vi "自定义模板.vi"() -> ()   [LabVIEW 2016]
uses:
  <vilib>/vision/Image Controls.llb/IMAQ Image.ctl
  <vilib>/vision/driver/IMAQdx.llb/IMAQdx Buffer Number Mode.ctl
  <vilib>/userdefined/High Color/IMAQdx.ctl
  <vilib>/vision/driver/IMAQdx.llb/IMAQdx Acquisition Mode.ctl
  <vilib>/vision/driver/NI_Vision_Acquisition_Software.lvlib
  <vilib>/vision/NI_Vision_Development_Module.lvlib
panel:
  in  "选项卡控件":enum32{"选项卡 1"}(tab)
  in  "导入图片":bool
  in  "保存按钮":bool
  in  "Stop":bool
  out "模板":T1(plugin-control)
  out "原图":T1(plugin-control)
  out "字符串":string="等待PLC端触发信号"
  in  "PLC触发拍照":bool
  # "自定义模板界面"
  # "1、点击导入图片选择原图.PNG"
  # "2、在原图中按住鼠标左键框选自定义模板（框选中间的圆形孔），选择完成后松开左键"
  # "3、模板中显示框选的模板，如不满意重新第二步骤"
  # "4、点击保存，在对话框中选择模板.PNG进行覆盖"
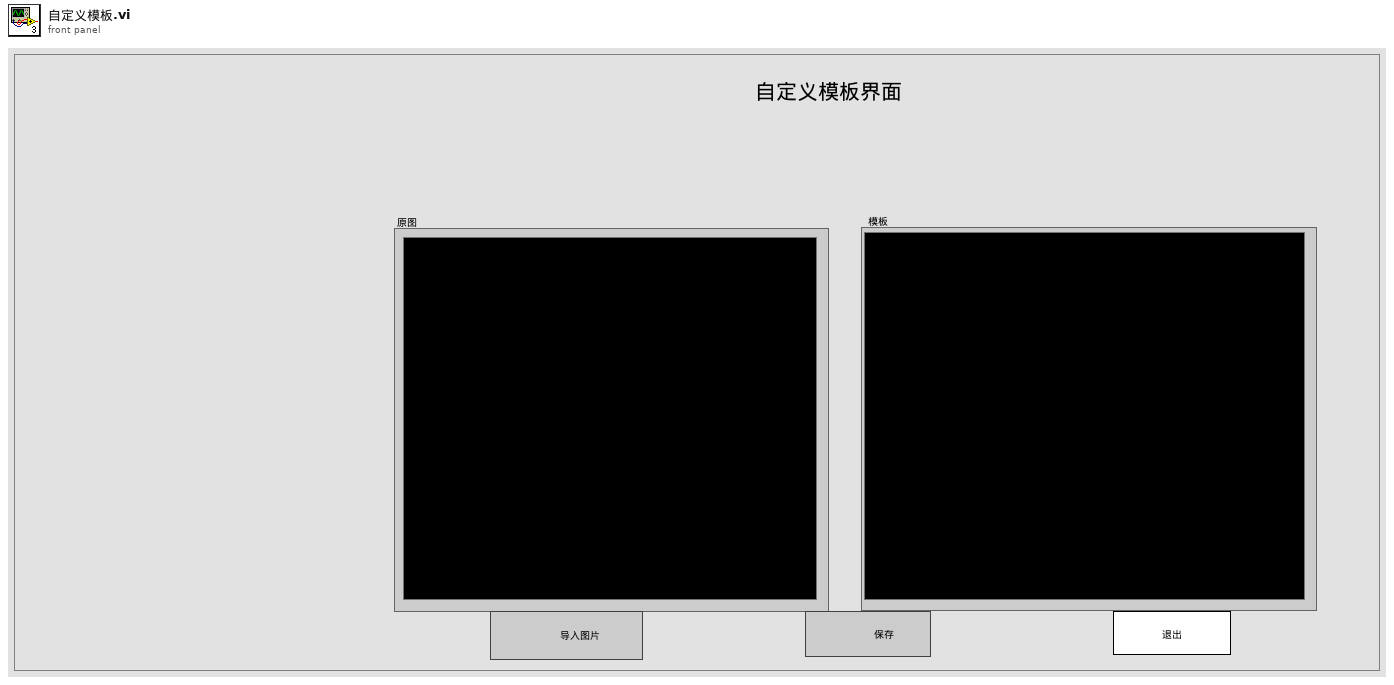
[diagram p1: front panel]
types:
  T1 = typedef "IMAQ Image.ctl" = refnum<image>
  T2 = typedef "建模板.ctl" = enum16{"等待", "拍照", "导入图片", "画模板", "保存模板", "左移", "右移", "上移", "下移", "旋转", "左右拉伸", "上下拉伸", "刷新图片", "保存参数", "退出"}
  T3 = enum8{"Enabled", "Disabled", "Disabled and Grayed Out"}
  T4 = typedef "Image Type" = u32
  T5 = cluster{"Zoom Tool":bool, "Selection Tool":bool, "Pan Tool":bool, "Point Tool":bool, "Line Tool":bool, "Rectangle Tool":bool, "Rotated Rectangle Tool":bool, "Polyline Tool":bool, "Polygon Tool":bool, "Freehand Tool":bool, "Closed Freehand Tool":bool, "Ellipse Tool":bool, "Annulus Tool":bool}
  T6 = typedef "NI_Vision_Acquisition_Software.lvlib/IMAQdx Acquisition Mode.ctl" = enum32{"One Shot", "Continuous"}
  T7 = typedef "IMAQdx.ctl" = refnum<k21>
  T8 = typedef "NI_Vision_Acquisition_Software.lvlib/IMAQdx Buffer Number Mode.ctl" = enum32{"Next", "Last", "Buffer Number", "Every", "Last New"}
  T9 = cluster{"Match Mode":u16, "Number of Matches Requested":i32, "Minimum Match Score":sgl, "SubPixel Accuracy":bool, "Rotation Angle Ranges":cluster{"Start":sgl, "End":sgl}[], "Show Search Area":bool, "Show Result":bool}
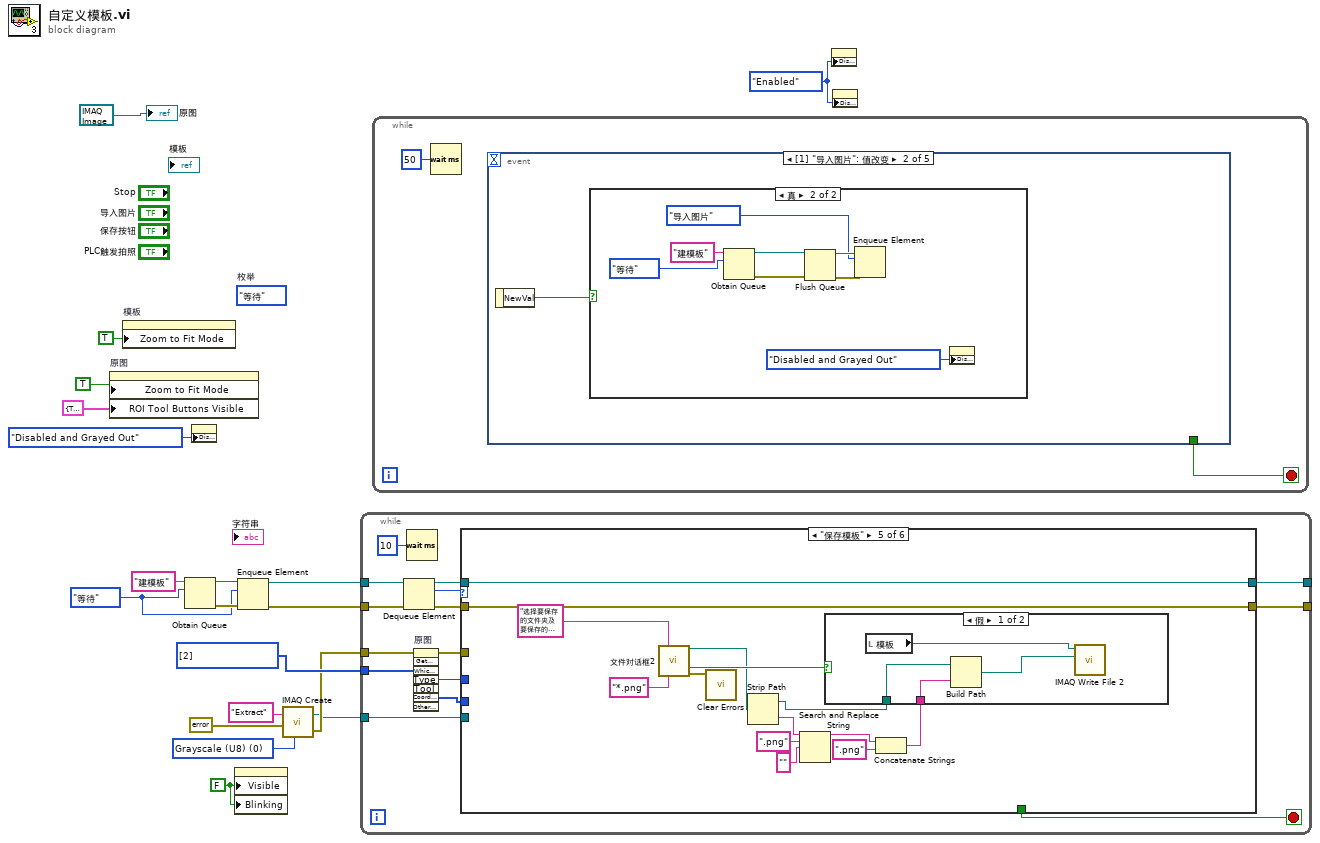
[diagram p0: block diagram]
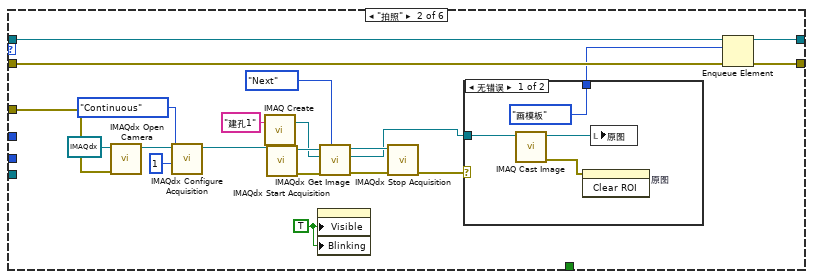
[diagram p3: hidden frame]
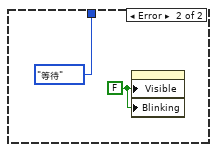
[diagram p4: hidden frame]
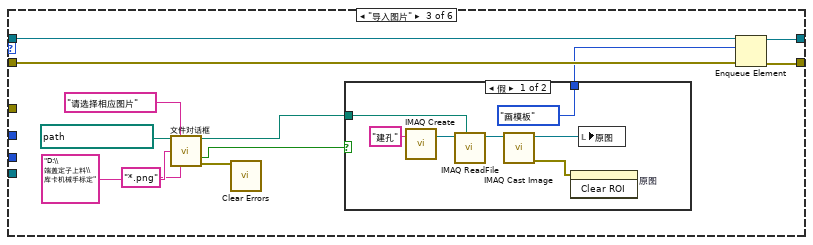
[diagram p5: hidden frame]
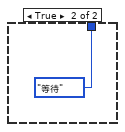
[diagram p6: hidden frame]
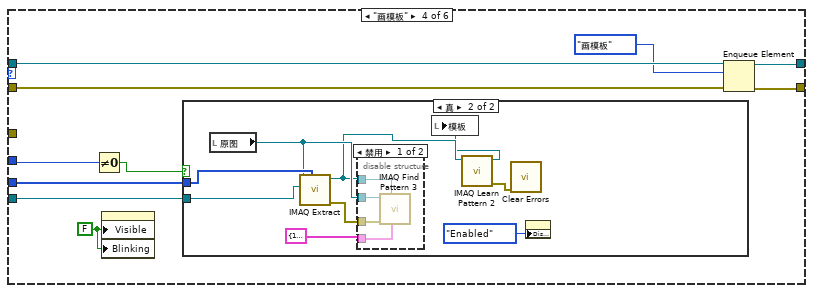
[diagram p7: hidden frame]
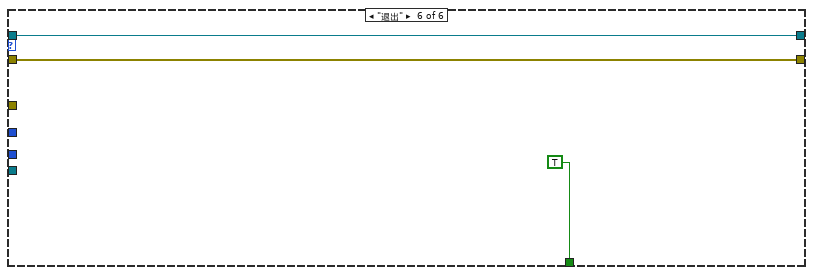
[diagram p11: hidden frame]
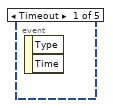
[diagram p12: hidden frame]
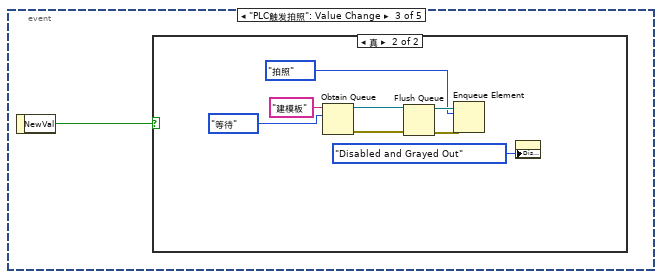
[diagram p14: hidden frame]
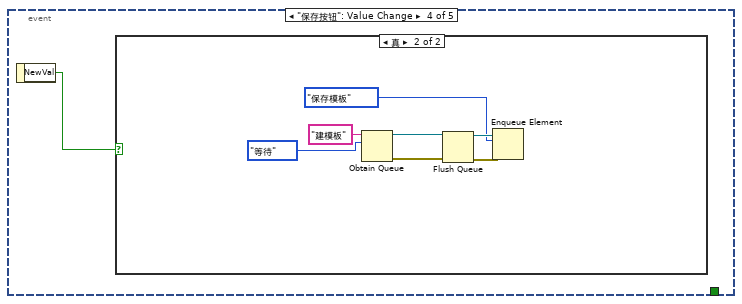
[diagram p16: hidden frame]
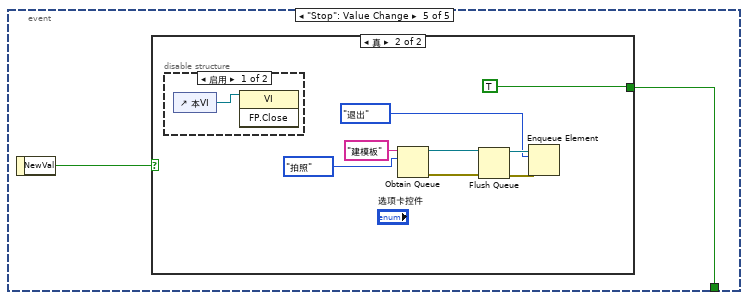
[diagram p18: hidden frame]
diagram:
  (unwired) 建模板."等待"  # 枚举
  w1 = FALSE ("可见")
  w2 = T3."Enabled" ("禁用")
  w3 = T4 0 items=["Grayscale (U8)", "Grayscale (I16)", "Grayscale (SGL)", "Complex (CSG)", "RGB (U32)", "HSL (U32)", "RGB (U64)", "Grayscale (U16)"] ("Image Type")
  w11 = i32[] [2] items=["No  event", "Click event", "Draw event", "Move event", "Size event", "Scroll event", "Activate event", "Close event", "Double click event"] ("Events list (all)")
  w16 = 建模板."等待"
  n1 = property on="原图" class="ImageControl"("Zoom to Fit Mode"=TRUE, "ROI Tool Buttons Visible"=T5 {"Zoom Tool"=TRUE, "Selection Tool"=FALSE, "Pan Tool"=TRUE, "Point Tool"=FALSE, "Line Tool"=FALSE, "Rectangle Tool"=TRUE, "Rotated Rectangle Tool"=FALSE, "Polyline Tool"=FALSE, "Polygon Tool"=FALSE, "Freehand Tool"=FALSE, "Closed Freehand Tool"=FALSE, "Ellipse Tool"=FALSE, "Annulus Tool"=FALSE} ("ROI Tool Buttons Visible:All Elements")) -> ()  [unwired: 2 in, 2 out]
  n2 = property on="模板" class="ImageControl"("Zoom to Fit Mode"=TRUE) -> ()  [unwired: 2 in, 2 out]
  n3 = Obtain Queue(name (unnamed)="建模板" ("名称（未命名）"), element data type=w16) -> (queue out=w17:refnum<queue>, error out=w18:errorcluster)  [unwired: 3 in, 1 out]
  n4 = property on="保存按钮" class="Bool (严格)"("DisabledEnum"=T3."Disabled and Grayed Out" ("禁用")) -> ()  [unwired: 2 in, 2 out]
  n5 = property on="字符串" class="Str"("Visible"=w1, "Blinking"=w1) -> ()  [unwired: 2 in, 2 out]
  n6 = Enqueue Element(queue=w17, element=w16, error in (no error)=w18) -> (queue out=w15:refnum<queue>, error out=w14:errorcluster)  [unwired: 1 in, 1 out]
  n7 = call "IMAQ Create"("Image Name"="Extract", "Image Type"=w3, "error in (no error)"=errorcluster {"status"=FALSE, "code"=0, "source"=""}) -> ("New Image"=w9:T1, "error out"=w10:errorcluster)  [unwired: 1 in, 1 out]
  n8 = while {
    tunnel: w15 -> [w34]
    tunnel: w14 -> [w33]
    tunnel: [w31] -> _
    tunnel: [w29] -> _
    tunnel: w11 -> [w27]
    tunnel: w10 -> [w25]
    tunnel: w9 -> [w23]
    stop <- w22 stop-if-true
    n9 = Dequeue Element(queue=w34, error in (no error)=w33) -> (queue out=w30:refnum<queue>, element=w32:T2, error out=w28:errorcluster)  [unwired: 1 in, 1 out]
    n10 = Wait (ms)(milliseconds to wait=u32 10 ("等待时间（毫秒）")) -> ()  [unwired: 1 out]
    n11 = invoke on="原图" class="ImageControl" method="Get Last Event"(error in=w25, "Which Events"=w27) -> (error out=w24:errorcluster, "Type"=w26:i32, "Coordinates"=w20:i32[])  [unwired: 6 in, 5 out]
    n12 = case shown="\"保存模板\"" w32 {
      tunnel: [w36 w57 w69 w93 w120 w127] -> w31
      tunnel: w30 -> [w36 w55 w71 w91 w120 w127]
      tunnel: [w35 w56 w68 w92 w119 w126] -> w29
      tunnel: w28 -> [w35 w54 w70 w87 w119 w126]
      tunnel: w26 -> [_ _ _ w86 _ _]
      tunnel: w24 -> [_ w42 _ _ _ _]
      tunnel: w23 -> [_ _ _ w90 _ _]
      tunnel: [_ _ _ _ _ TRUE] -> w22
      tunnel: w20 -> [_ _ _ w89 _ _]
      frame "等待", Default {
      }
      frame "拍照" {
        w48 = TRUE ("可见")
        n13 = call <vilib>:"IMAQdx Open Camera.vi"("error in"=w42, "Session In"=T7 refnum) -> ("Session Out"=w40:T7)  [unwired: 8 in, 1 out]
        n14 = call <vilib>:"IMAQdx Configure Acquisition.vi"("Number of Buffers"=u32 1, "Continuous?"=IMAQdx_Acquisition_Mode."Continuous", "Session In"=w40) -> ("Session Out"=w39:T7)  [unwired: 7 in, 1 out]
        n15 = call "IMAQ Create"("Image Name"="建孔1") -> ("New Image"=w50:T1)  [unwired: 4 in, 1 out]
        n16 = call <vilib>:"IMAQdx Start Acquisition.vi"("Session In"=w39) -> ("error out"=w47:errorcluster, "Session Out"=w52:T7)  [unwired: 9 in]
        n17 = property on="字符串" class="Str"("Visible"=w48, "Blinking"=w48) -> ()  [unwired: 2 in, 2 out]
        n18 = call <vilib>:"IMAQdx Get Image.vi"("Buffer Number Mode (Next)"=IMAQdx_Buffer_Number_Mode."Next", "error in"=w47, "Image In"=w50, "Session In"=w52) -> ("error out"=w46:errorcluster, "Image Out"=w43:T1, "Session Out"=w45:T7)  [unwired: 4 in, 1 out]
        n19 = call <vilib>:"IMAQdx Stop Acquisition.vi"("error in"=w46, "Session In"=w45) -> ("error out"=w44:errorcluster)  [unwired: 8 in, 1 out]
        n20 = case shown="无错误" w44 {
          tunnel: [建模板."画模板" 建模板."等待"] -> w53
          tunnel: w43 -> [w58 _]
          frame No Error {
            n21 = call "IMAQ Cast Image"("Image Src"=w58) -> ("error out"=w61:errorcluster, "Image Dst Out"=w60:T1)  [unwired: 9 in]
            n22 = invoke on="原图" class="ImageControl" method="Clear ROI"(error in=w61) -> ()  [unwired: 2 in, 3 out]
            n23 = local write "原图"(w60) -> ()
          }
          frame Error {
            w62 = FALSE ("可见")
            n24 = property on="字符串" class="Str"("Visible"=w62, "Blinking"=w62) -> ()  [unwired: 2 in, 2 out]
          }
        }
        n25 = Enqueue Element(queue=w55, element=w53, error in (no error)=w54) -> (queue out=w57:refnum<queue>, error out=w56:errorcluster)  [unwired: 1 in, 1 out]
      }
      frame "导入图片" {
        n26 = call "文件对话框"("start path"=path "D:/端盖定子上料/库卡机械手标定" ("File Path 3"), "prompt"="请选择相应图片", "default name"="D:\\端盖定子上料\\库卡机械手标定", "pattern (all files)"="*.png") -> ("selected path"=w66:path, "cancelled"=w72:bool, "error out"=w73:errorcluster)  [unwired: 8 in, 1 out]
        n27 = call <vilib>:"Clear Errors.vi"("error in (no error)"=w73) -> ()  [unwired: 5 in, 2 out]
        n28 = case shown="假" w72 {
          tunnel: [建模板."画模板" 建模板."等待"] -> w67
          tunnel: w66 -> [w77 _]
          frame False {
            n29 = call "IMAQ Create"("Image Name"="建孔") -> ("New Image"=w80:T1)  [unwired: 4 in, 1 out]
            n30 = call "IMAQ ReadFile"("File Path"=w77, "Image"=w80) -> ("Image Out"=w78:T1)  [unwired: 5 in, 4 out]
            n31 = call "IMAQ Cast Image"("Image Src"=w78) -> ("error out"=w82:errorcluster, "Image Dst Out"=w81:T1)  [unwired: 9 in]
            n32 = invoke on="原图" class="ImageControl" method="Clear ROI"(error in=w82) -> ()  [unwired: 2 in, 3 out]
            n33 = local write "原图"(w81) -> ()
          }
          frame True {
          }
        }
        n34 = Enqueue Element(queue=w71, element=w67, error in (no error)=w70) -> (queue out=w69:refnum<queue>, error out=w68:errorcluster)  [unwired: 1 in, 1 out]
      }
      frame "画模板" {
        w84 = FALSE ("可见")
        n35 = Not Equal To 0?(x=w86) -> (x != 0?=w85:bool)
        n36 = property on="字符串" class="Str"("Visible"=w84, "Blinking"=w84) -> ()  [unwired: 2 in, 2 out]
        n37 = case shown="真" w85 {
          tunnel: w90 -> [_ w99]
          tunnel: w89 -> [_ w98]
          frame False {
          }
          frame True {
            n38 = local read "原图"() -> (w97:T1)
            n39 = call "IMAQ Extract"("Optional Rectangle"=w98, "Image Dst"=w99, "Image Src"=w97) -> ("error out"=w102:errorcluster, "Image Dst Out"=w96:T1)  [unwired: 3 in, 4 out]
            n40 = disable-structure shown="禁用" {
              disable-tunnel: w102 -> [w106 _]
              disable-tunnel: w96 -> [w104 _]
              disable-tunnel: T9 {"Match Mode"=1, "Number of Matches Requested"=1, "Minimum Match Score"=500.0, "SubPixel Accuracy"=TRUE, "Rotation Angle Ranges"=[], "Show Search Area"=FALSE, "Show Result"=TRUE} ("Settings") -> [w105 _]
              disable-tunnel: w97 -> [w103 _]
              frame Disabled {
                n41 = call "IMAQ Find Pattern 3"("Settings"=w105, "Template"=w104, "error in (no error)"=w106, "Image"=w103) -> ()  [unwired: 2 in, 6 out]
              }
              frame Enabled {
              }
            }
            n42 = call "IMAQ Learn Pattern 2"("Image"=w96) -> ("error out"=w94:errorcluster, "Template Image Out"=w95:T1)  [unwired: 9 in]
            n43 = local write "模板"(w95) -> ()
            n44 = call <vilib>:"Clear Errors.vi"("error in (no error)"=w94) -> ()  [unwired: 5 in, 2 out]
            n45 = property on="保存按钮" class="Bool (严格)"("DisabledEnum"=T3."Enabled" ("禁用")) -> ()  [unwired: 2 in, 2 out]
          }
        }
        n46 = Enqueue Element(queue=w91, element=建模板."画模板", error in (no error)=w87) -> (queue out=w93:refnum<queue>, error out=w92:errorcluster)  [unwired: 1 in, 1 out]
      }
      frame "保存模板" {
        n47 = call "文件对话框2"("prompt"="选择要保存的文件夹及要保存的图片名", "pattern (all files)"="*.png") -> ("selected path"=w116:path, "cancelled"=w117:bool, "error out"=w118:errorcluster)  [unwired: 10 in, 1 out]
        n48 = call <vilib>:"Clear Errors.vi"("error in (no error)"=w118) -> ()  [unwired: 5 in, 2 out]
        n49 = Strip Path(path=w116) -> (stripped path=w113:path, name=w108:string)
        n50 = Search and Replace String(input string=w108, search string=".png" ("搜索字符串"), replace string="" ("替换字符串(\"\")")) -> (result string=w112:string)  [unwired: 5 in, 3 out]
        n51 = Concatenate Strings(w112, ".png" ("字符串")) -> (w114:string)
        n52 = case shown="假" w117 {
          tunnel: w113 -> [w124 _]
          tunnel: w114 -> [w123 _]
          frame False {
            n53 = local read "模板"() -> (w121:T1)
            n54 = Build Path(base path=w124, name or relative path=w123) -> (appended path=w122:path)
            n55 = call-poly "IMAQ Write File 2"("File Path"=w122, "Image"=w121) -> ()  [unwired: 8 in, 2 out]
          }
          frame True {
          }
        }
      }
      frame "退出" {
      }
    }
  }
  n56 = while {
    stop <- w128 stop-if-true
    n57 = Wait (ms)(milliseconds to wait=u32 50 ("等待时间（毫秒）")) -> ()  [unwired: 1 out]
    n58 = event shown="[1] \"导入图片\": 值改变" {
      selector: _ -> [_ _ _ _ _]
      dyn-events: _ -> [_ _ _ _ _]
      timeout: _ -> [_ _ _ _ _]
      tunnel: [_ _ _ _ w156] -> w128
      event Timeout {
        n59 = event-data() -> ()  [unwired: 1 in, 2 out]
      }
      event "导入图片": Value Change {
        n60 = event-data() -> ("NewVal"=w130:bool)  [unwired: 1 in]
        n61 = case shown="真" w130 {
          frame False {
          }
          frame True {
            n62 = Obtain Queue(name (unnamed)="建模板" ("名称（未命名）"), element data type=建模板."等待") -> (queue out=w136:refnum<queue>, error out=w135:errorcluster)  [unwired: 3 in, 1 out]
            n63 = Flush Queue(queue=w136, error in (no error)=w135) -> (queue out=w134:refnum<queue>, error out=w133:errorcluster)  [unwired: 1 out]
            n64 = Enqueue Element(queue=w134, element=建模板."导入图片", error in (no error)=w133) -> ()  [unwired: 1 in, 3 out]
            n65 = property on="保存按钮" class="Bool (严格)"("DisabledEnum"=T3."Disabled and Grayed Out" ("禁用")) -> ()  [unwired: 2 in, 2 out]
          }
        }
      }
      event "PLC触发拍照": Value Change {
        n66 = event-data() -> ("NewVal"=w139:bool)  [unwired: 1 in]
        n67 = case shown="真" w139 {
          frame False {
          }
          frame True {
            n68 = Obtain Queue(name (unnamed)="建模板" ("名称（未命名）"), element data type=建模板."等待") -> (queue out=w145:refnum<queue>, error out=w144:errorcluster)  [unwired: 3 in, 1 out]
            n69 = Flush Queue(queue=w145, error in (no error)=w144) -> (queue out=w143:refnum<queue>, error out=w142:errorcluster)  [unwired: 1 out]
            n70 = Enqueue Element(queue=w143, element=建模板."拍照", error in (no error)=w142) -> ()  [unwired: 1 in, 3 out]
            n71 = property on="保存按钮" class="Bool (严格)"("DisabledEnum"=T3."Disabled and Grayed Out" ("禁用")) -> ()  [unwired: 2 in, 2 out]
          }
        }
      }
      event "保存按钮": Value Change {
        n72 = event-data() -> ("NewVal"=w148:bool)  [unwired: 1 in]
        n73 = case shown="真" w148 {
          frame False {
          }
          frame True {
            n74 = Obtain Queue(name (unnamed)="建模板" ("名称（未命名）"), element data type=建模板."等待") -> (queue out=w153:refnum<queue>, error out=w152:errorcluster)  [unwired: 3 in, 1 out]
            n75 = Flush Queue(queue=w153, error in (no error)=w152) -> (queue out=w151:refnum<queue>, error out=w150:errorcluster)  [unwired: 1 out]
            n76 = Enqueue Element(queue=w151, element=建模板."保存模板", error in (no error)=w150) -> ()  [unwired: 1 in, 3 out]
          }
        }
      }
      event "Stop": Value Change {
        n77 = event-data() -> ("NewVal"=w157:bool)  [unwired: 1 in]
        n78 = case shown="真" w157 {
          tunnel: [_ TRUE] -> w156
          frame False {
          }
          frame True {
            n79 = disable-structure shown="启用" {
              frame Enabled {
                n80 = control-ref of="本VI"() -> (w166:refnum<vi>)
                n81 = invoke class="VI" method="FP.Close"(reference=w166) -> ()  [unwired: 2 in, 3 out]
              }
              frame Disabled {
              }
            }
            n82 = Obtain Queue(name (unnamed)="建模板" ("名称（未命名）"), element data type=建模板."拍照") -> (queue out=w163:refnum<queue>, error out=w162:errorcluster)  [unwired: 3 in, 1 out]
            n83 = Flush Queue(queue=w163, error in (no error)=w162) -> (queue out=w161:refnum<queue>, error out=w160:errorcluster)  [unwired: 1 out]
            n84 = Enqueue Element(queue=w161, element=建模板."退出", error in (no error)=w160) -> ()  [unwired: 1 in, 3 out]
          }
        }
      }
    }
  }
  n85 = property on="导入图片" class="Bool (严格)"("DisabledEnum"=w2) -> ()  [unwired: 2 in, 2 out]
  n86 = property on="PLC触发拍照" class="Bool (严格)"("DisabledEnum"=w2) -> ()  [unwired: 2 in, 2 out]
  "原图" <- T1 refnum ("Image 2")
